vi "Arrange Control Labels.vi"(8 "error in (no error)":errorcluster, 11 "vi path":path) -> (0 "error out":errorcluster)   [LabVIEW 2023]
uses:
  <vilib>/Utility/traverseref.llb/TRef TravTarget.ctl
  <vilib>/Utility/QuickDropSupport/QuickDrop Plugin Data ver1.ctl
  <vilib>/Utility/traverseref.llb/VI Scripting - Traverse.lvlib
panel:
  in  "Combo Box":string(combo)
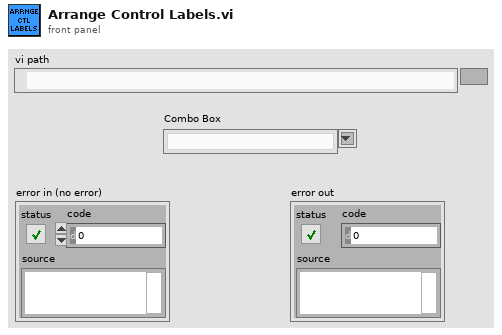
[diagram p1: front panel]
types:
  T1 = typedef "QuickDrop Plugin Data ver1.ctl" = cluster{"FP.IsFrontMost?":bool, "Project VI Path":path, "Palette Object Name":string}
  T2 = typedef "TRef TravTarget.ctl" = enum16{"FP", "BD", "Other"}
  T3 = typedef "LVPositionTypeDef.ctl" = cluster{"Left":i32, "Top":i32}
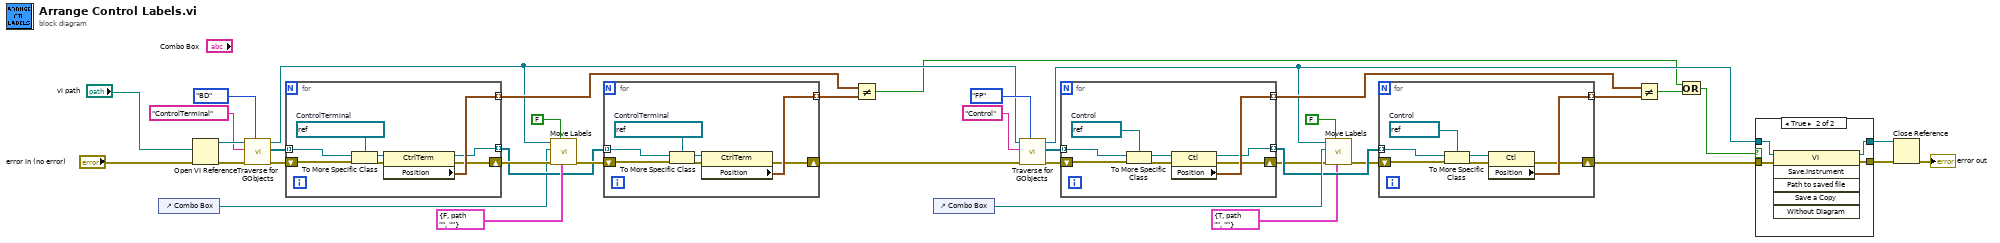
[diagram p0: block diagram]
diagram:
  n1 = control-ref of="Combo Box"() -> (w20:refnum<vi>)
  n2 = Open VI Reference(vi path="vi path", error in (no error)="error in (no error)") -> (vi reference=w32:refnum<vi>, error out=w33:errorcluster)  [unwired: 4 in]
  n3 = call <vilib>:"Traverse for GObjects.vi"("Traverse Target"=TRef_TravTarget."BD", "error in (no error)"=w33, "Class Name"="ControlTerminal", "VI Refnum"=w32) -> ("error out"=w30:errorcluster, "References"=w29:refnum<vi>[], "dup VI Refnum"=w7:refnum<vi>)  [unwired: 4 in, 1 out]
  n4 = for {
    tunnel: w29 -> [w46] mode=indexing
    shift-right: [w40] -> w25
    shift-left: w30 -> [w42]
    tunnel: [w41] -> w21 mode=indexing
    tunnel: [w39] -> w23 mode=indexing
    w45 = refnum<vi> refnum  # ControlTerminal
    n5 = To More Specific Class(target class=w45, reference=w46, error in=w42) -> (specific class reference=w44:refnum<vi>, error out=w43:errorcluster)
    n6 = property class="CtrlTerm"(reference=w44, error in=w43) -> (reference out=w39:refnum<vi>, error out=w40:errorcluster, "Position"=w41:T3)
  }
  n7 = call <resource>:"Move Labels.vi"("Variant in"=T1 {"FP.IsFrontMost?"=FALSE, "Project VI Path"=path "", "Palette Object Name"=""} ("Quick Drop Plugin Data"), "Shift Pressed?"=FALSE, "error in (no error)"=w25, "QD Combo Box Ref"=w20, "QD Launch VI Ref"=w7) -> ("error out"=w24:errorcluster)  [unwired: 5 in, 1 out]
  n8 = for {
    tunnel: w23 -> [w53] mode=indexing
    shift-right: [w47] -> w8
    shift-left: w24 -> [w49]
    tunnel: [w48] -> w22 mode=indexing
    w52 = refnum<vi> refnum  # ControlTerminal
    n9 = To More Specific Class(target class=w52, reference=w53, error in=w49) -> (specific class reference=w51:refnum<vi>, error out=w50:errorcluster)
    n10 = property class="CtrlTerm"(reference=w51, error in=w50) -> (error out=w47:errorcluster, "Position"=w48:T3)  [unwired: 1 out]
  }
  n11 = Not Equal?(x=w21, y=w22) -> (x != y?=w2:bool)
  n12 = control-ref of="Combo Box"() -> (w19:refnum<vi>)
  n13 = call <vilib>:"Traverse for GObjects.vi"("Traverse Target"=TRef_TravTarget."FP", "error in (no error)"=w8, "Class Name"="Control", "VI Refnum"=w7) -> ("error out"=w10:errorcluster, "References"=w11:refnum<vi>[], "dup VI Refnum"=w4:refnum<vi>)  [unwired: 4 in, 1 out]
  n14 = for {
    tunnel: w11 -> [w61] mode=indexing
    shift-right: [w55] -> w15
    shift-left: w10 -> [w57]
    tunnel: [w56] -> w6 mode=indexing
    tunnel: [w54] -> w17 mode=indexing
    w60 = refnum<vi> refnum  # Control
    n15 = To More Specific Class(target class=w60, reference=w61, error in=w57) -> (specific class reference=w59:refnum<vi>, error out=w58:errorcluster)
    n16 = property class="Ctl"(reference=w59, error in=w58) -> (reference out=w54:refnum<vi>, error out=w55:errorcluster, "Position"=w56:T3)
  }
  n17 = call <resource>:"Move Labels.vi"("Variant in"=T1 {"FP.IsFrontMost?"=TRUE, "Project VI Path"=path "", "Palette Object Name"=""} ("Quick Drop Plugin Data"), "Shift Pressed?"=FALSE, "error in (no error)"=w15, "QD Combo Box Ref"=w19, "QD Launch VI Ref"=w4) -> ("error out"=w16:errorcluster)  [unwired: 5 in, 1 out]
  n18 = for {
    tunnel: w17 -> [w68] mode=indexing
    shift-right: [w62] -> w5
    shift-left: w16 -> [w64]
    tunnel: [w63] -> w18 mode=indexing
    w67 = refnum<vi> refnum  # Control
    n19 = To More Specific Class(target class=w67, reference=w68, error in=w64) -> (specific class reference=w66:refnum<vi>, error out=w65:errorcluster)
    n20 = property class="Ctl"(reference=w66, error in=w65) -> (error out=w62:errorcluster, "Position"=w63:T3)  [unwired: 1 out]
  }
  n21 = Not Equal?(x=w6, y=w18) -> (x != y?=w3:bool)
  n22 = Or(x=w2, y=w3) -> (x .or. y?=w1:bool)
  n23 = case shown="True" w1 {
    tunnel: [w70 w74] -> w35
    tunnel: [w69 w73] -> w34
    tunnel: w5 -> [w70 w72]
    tunnel: w4 -> [w69 w71]
    frame False {
    }
    frame True {
      n24 = invoke class="VI" method="Save.Instrument"(reference=w71, error in=w72) -> (reference out=w73:refnum<vi>, error out=w74:errorcluster)  [unwired: 4 in, 4 out]
    }
  }
  n25 = Close Reference(reference=w34, error in (no error)=w35) -> (error out=→"error out":errorcluster)
